vi "temptofinalbuffer.vi"(0 "current average":dbl) -> ()   [LabVIEW 2013]
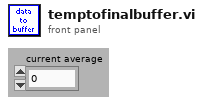
[diagram p1: front panel]
types:
  T1 = cluster{"Xpixels":i32, "Vx-min ref":dbl, "Vx-max ref":dbl, "Ypixels":i32, "Vy-min ref":dbl, "Vy-max ref":dbl, "srate":dbl, "type":string, "date":string, "time":string, "Colormap":u16, "square pixels":bool, "square matrix":bool, "Xpixels Img":i32, "Vx-min Img":dbl, "VX-max Img":dbl, "Ypixels Img":i32, "Vy-min Img":dbl, "Vy-max Img ":dbl, "autoshutter":bool, "P":dbl, "sAOxy":i32, "finite":bool, "cont":bool, "wavdet":bool, "measpoints":i32, "avpp":i32, "bufferAO":i32, "bufferAI":i32, "CH1":bool, "CH2":bool, "X":bool, "Y":bool, "timeout":dbl, "starttick":u32, "waveform":path, "Vy-ref":dbl, "Vx-ref":dbl, "refreshrate":dbl, "refreshbuffer":i32, "tt_cycles":i32, "motorref":refnum<k7>, "mirrorswitch":refnum<k7>, "sample mode":i32, "Ip":bool, "Vp":bool, "sampletreshold":dbl, "maxbufferAI":i32, "Angle Img":dbl}
  T2 = cluster{"CH1 AI":tag, "CH1 CI":tag, "CH2 AI":tag, "CH2 CI":tag, "AI X":tag, "AI Y":tag, "AO X-Y":tag, "CH1ST":bool, "CH2ST":bool, "Sigcase":i16, "StageS":i32, "StageL":i32, "data dir":path, "Vp":tag, "Ip":tag, "AO CWlaser":tag, "AO VtoP":tag, "shutter":tag, "488":tag, "532":tag, "640":tag}
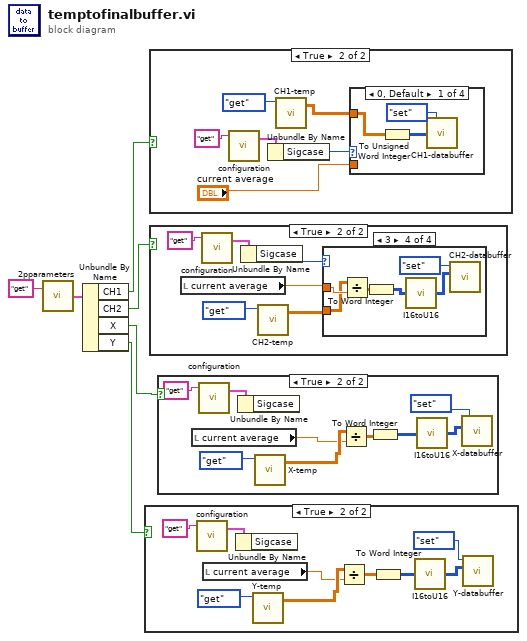
[diagram p0: block diagram]
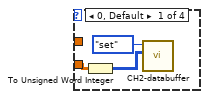
[diagram p5: hidden frame]
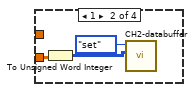
[diagram p6: hidden frame]
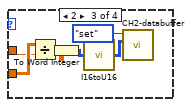
[diagram p7: hidden frame]
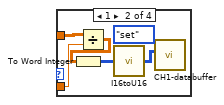
[diagram p9: hidden frame]
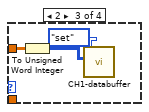
[diagram p10: hidden frame]
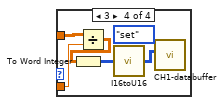
[diagram p11: hidden frame]
diagram:
  n1 = call "2pparameters.vi"("command"="get") -> ("Params out"=w2:T1)  [unwired: 1 in]
  n2 = Unbundle By Name(w2) -> ("CH1"=w3:bool, "CH2"=w4:bool, "X"=w5:bool, "Y"=w6:bool)
  n3 = case shown="True" w6 {
    frame False {
    }
    frame True {
      n4 = call "configuration.vi"("command"="get") -> ("config out"=w14:T2)  [unwired: 2 in, 1 out]
      n5 = local read "current average"() -> (w7:dbl)
      n6 = Unbundle By Name(w14) -> ()  [unwired: 1 out]
      n7 = call "Y-temp.vi"("command"=enum16{"get", "set", "clear", "add row"}."get") -> ("array out"=w12:sgl[][])  [unwired: 3 in, 1 out]
      n8 = Divide(x=w12, y=w7) -> (x/y=w8:dbl[][])
      n9 = To Word Integer(number=w8) -> (16bit integer=w9:i16[][])
      n10 = call "I16toU16.vi"("I16"=w9) -> ("U16"=w10:u16[][])
      n11 = call "Y-databuffer.vi"("array in"=w10, "command"=enum16{"get", "set", "clear", "add row"}."set") -> ()  [unwired: 2 in, 2 out]
    }
  }
  n12 = case shown="True" w3 {
    frame False {
    }
    frame True {
      n13 = call "configuration.vi"("command"="get") -> ("config out"=w20:T2)  [unwired: 2 in, 1 out]
      n14 = Unbundle By Name(w20) -> ("Sigcase"=w19:i16)
      n15 = call "CH1-temp.vi"("command"=enum16{"get", "set", "clear", "add row"}."get") -> ("array out"=w17:sgl[][])  [unwired: 3 in, 1 out]
      n16 = case shown="0, Default" w19 {
        tunnel: "current average" -> [_ w30 _ w39]
        tunnel: w17 -> [w23 w29 w32 w38]
        frame 0, Default {
          n17 = To Unsigned Word Integer(number=w23) -> (unsigned 16bit integer=w24:u16[][])
          n18 = call "CH1-databuffer.vi"("array in"=w24, "command"=enum16{"get", "set", "clear", "add row"}."set") -> ()  [unwired: 2 in, 2 out]
        }
        frame 1 {
          n19 = Divide(x=w29, y=w30) -> (x/y=w26:dbl[][])
          n20 = To Word Integer(number=w26) -> (16bit integer=w27:i16[][])
          n21 = call "I16toU16.vi"("I16"=w27) -> ("U16"=w28:u16[][])
          n22 = call "CH1-databuffer.vi"("array in"=w28, "command"=enum16{"get", "set", "clear", "add row"}."set") -> ()  [unwired: 2 in, 2 out]
        }
        frame 2 {
          n23 = To Unsigned Word Integer(number=w32) -> (unsigned 16bit integer=w33:u16[][])
          n24 = call "CH1-databuffer.vi"("array in"=w33, "command"=enum16{"get", "set", "clear", "add row"}."set") -> ()  [unwired: 2 in, 2 out]
        }
        frame 3 {
          n25 = Divide(x=w38, y=w39) -> (x/y=w35:dbl[][])
          n26 = To Word Integer(number=w35) -> (16bit integer=w36:i16[][])
          n27 = call "I16toU16.vi"("I16"=w36) -> ("U16"=w37:u16[][])
          n28 = call "CH1-databuffer.vi"("array in"=w37, "command"=enum16{"get", "set", "clear", "add row"}."set") -> ()  [unwired: 2 in, 2 out]
        }
      }
    }
  }
  n29 = case shown="True" w4 {
    frame False {
    }
    frame True {
      n30 = local read "current average"() -> (w40:dbl)
      n31 = call "configuration.vi"("command"="get") -> ("config out"=w44:T2)  [unwired: 2 in, 1 out]
      n32 = Unbundle By Name(w44) -> ("Sigcase"=w43:i16)
      n33 = call "CH2-temp.vi"("command"=enum16{"get", "set", "clear", "add row"}."get") -> ("array out"=w41:sgl[][])  [unwired: 3 in, 1 out]
      n34 = case shown="3" w43 {
        tunnel: w40 -> [_ _ w56 w63]
        tunnel: w41 -> [w46 w49 w57 w62]
        frame 0, Default {
          n35 = To Unsigned Word Integer(number=w46) -> (unsigned 16bit integer=w48:u16[][])
          n36 = call "CH2-databuffer.vi"("array in"=w48, "command"=enum16{"get", "set", "clear", "add row"}."set") -> ()  [unwired: 2 in, 2 out]
        }
        frame 1 {
          n37 = To Unsigned Word Integer(number=w49) -> (unsigned 16bit integer=w51:u16[][])
          n38 = call "CH2-databuffer.vi"("array in"=w51, "command"=enum16{"get", "set", "clear", "add row"}."set") -> ()  [unwired: 2 in, 2 out]
        }
        frame 2 {
          n39 = Divide(x=w57, y=w56) -> (x/y=w52:dbl[][])
          n40 = To Word Integer(number=w52) -> (16bit integer=w53:i16[][])
          n41 = call "I16toU16.vi"("I16"=w53) -> ("U16"=w55:u16[][])
          n42 = call "CH2-databuffer.vi"("array in"=w55, "command"=enum16{"get", "set", "clear", "add row"}."set") -> ()  [unwired: 2 in, 2 out]
        }
        frame 3 {
          n43 = Divide(x=w62, y=w63) -> (x/y=w58:dbl[][])
          n44 = To Word Integer(number=w58) -> (16bit integer=w60:i16[][])
          n45 = call "I16toU16.vi"("I16"=w60) -> ("U16"=w61:u16[][])
          n46 = call "CH2-databuffer.vi"("array in"=w61, "command"=enum16{"get", "set", "clear", "add row"}."set") -> ()  [unwired: 2 in, 2 out]
        }
      }
    }
  }
  n47 = case shown="True" w5 {
    frame False {
    }
    frame True {
      n48 = local read "current average"() -> (w64:dbl)
      n49 = call "configuration.vi"("command"="get") -> ("config out"=w71:T2)  [unwired: 2 in, 1 out]
      n50 = Unbundle By Name(w71) -> ()  [unwired: 1 out]
      n51 = call "X-temp.vi"("command"=enum16{"get", "set", "clear", "add row"}."get") -> ("array out"=w69:sgl[][])  [unwired: 3 in, 1 out]
      n52 = Divide(x=w69, y=w64) -> (x/y=w65:dbl[][])
      n53 = To Word Integer(number=w65) -> (16bit integer=w66:i16[][])
      n54 = call "I16toU16.vi"("I16"=w66) -> ("U16"=w68:u16[][])
      n55 = call "X-databuffer.vi"("array in"=w68, "command"=enum16{"get", "set", "clear", "add row"}."set") -> ()  [unwired: 2 in, 2 out]
    }
  }
